vi "Quiz1_TP059851_Sim Yoke Shin.vi"() -> ()   [LabVIEW 2020]
panel:
  out "Warning Signal":bool
  in  "Chermical rate\n(litres/second)":dbl(slide) scale=0.0..50.0
  in  "Temperature":dbl(slide) scale=0.0..100.0
  in  "Concentration":dbl(slide) scale=0.0..10.0
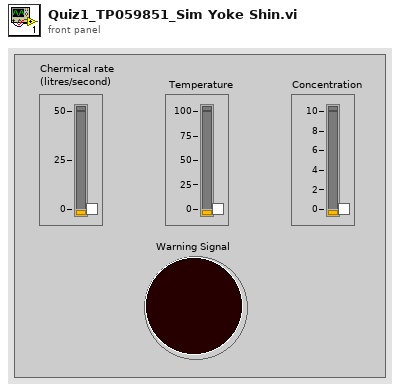
[diagram p1: front panel]
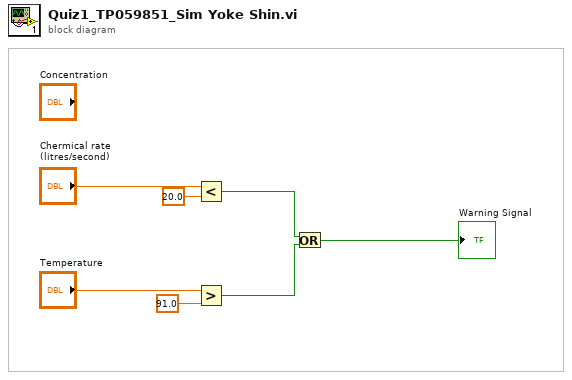
[diagram p0: block diagram]
diagram:
  n1 = Less?(x="Chermical rate\n(litres/second)", y=20.0) -> (x < y?=w3:bool)
  n2 = Greater?(x="Temperature", y=91.0) -> (0:w2:bool)
  n3 = Or(x=w3, y=w2) -> (x .or. y?=→"Warning Signal":bool)
